vi "使用子vi.vi"   [LabVIEW 2020]
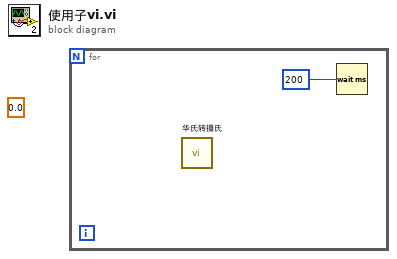
[diagram p0: block diagram]
diagram:
  (unwired) 0.0
  n1 = for {
    n2 = call "华氏转摄氏.vi"() -> ()  [unwired: 11 in, 1 out]
    n3 = Wait (ms)(milliseconds to wait=200) -> ()  [unwired: 1 out]
  }
